vi "FlowThroughNMR.vi"() -> ()   [LabVIEW 2021]
uses:
  <instrlib>/niFgen/niFgen.llb/niFgen Output Mode.ctl
  <vilib>/Utility/file.llb/Write Delimited Spreadsheet (DBL).vi
panel:
  in  "File Folder for Data":string
  out "size(s)":i32
  out "Numeric":dbl
  in  "Write Output to File?":bool=TRUE
  out "Averaged T2 Decay":waveform(dbl)(graph)={"t0"=timestamp(0 s since 1904-01-01), "dt"=0.0012610340479192938, "Y"=array[3965 elements]} caption="Waveform Graph"
  in  "Number of Scans":i32=8
  out "Signal Intensity (Integral)":dbl=0.6544283602926818 format="%0.4f"
  out "Scan Number":i32=8
  out "Final Larmor Frequency":dbl format="%#_10g"
  in  "Pulse Train File":path=path "C:/Users/localuser/OneDrive - University of South Carolina/NMR Research/MATLAB/6 us 90 Degree - 1.25ms Tau - 3965 Pulses.txt"
  in  "Initial Larmor Frequency":dbl=27410000.0 caption="Frequency" format="%.3p"
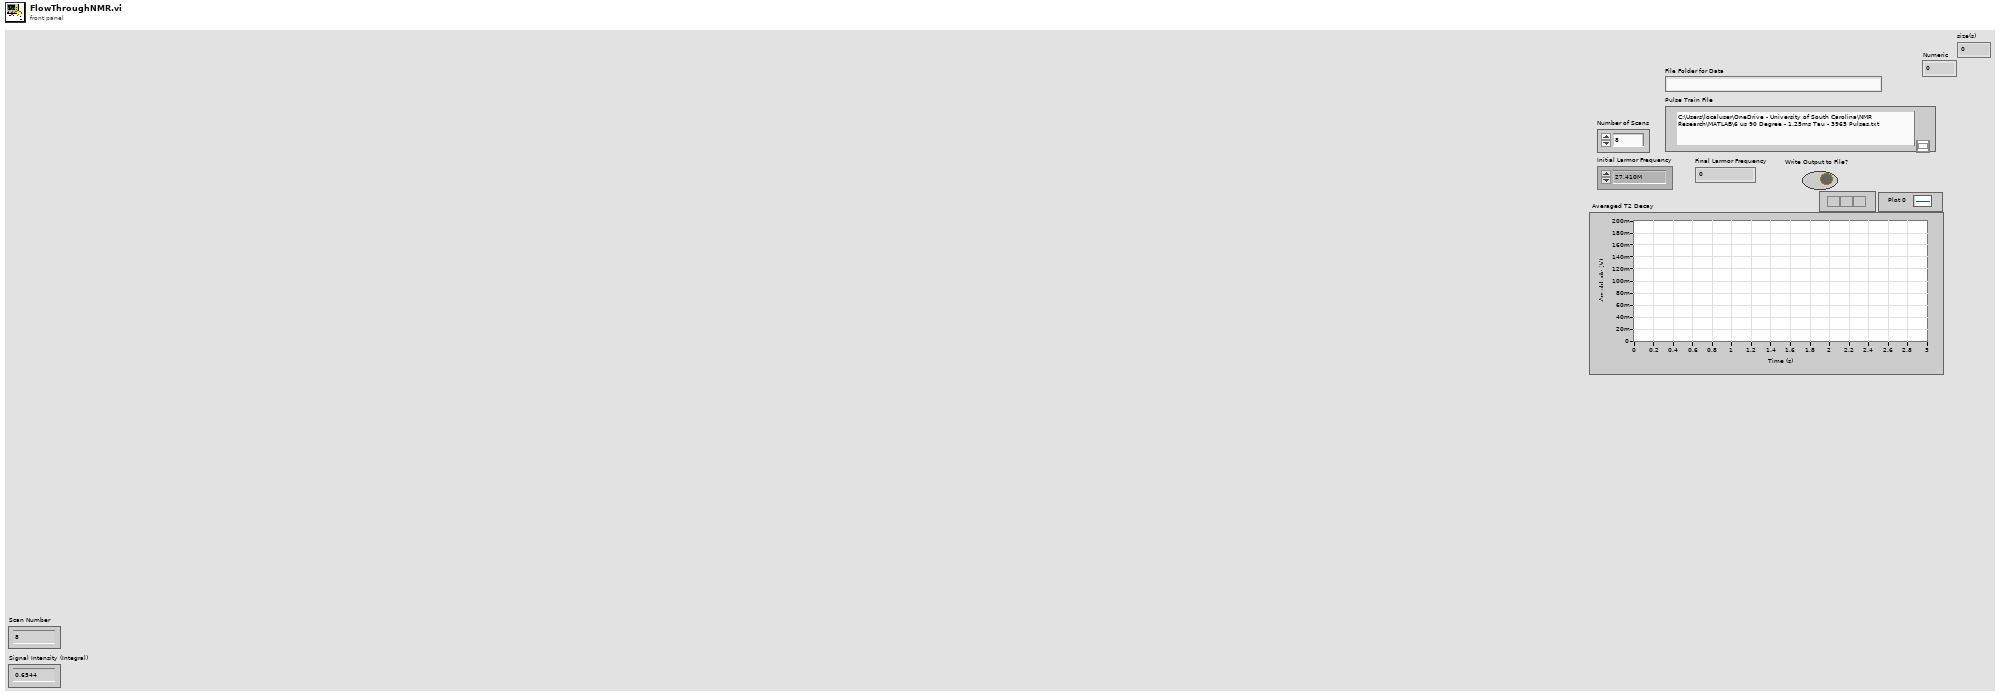
[diagram p1: front panel]
types:
  T1 = typedef "niFgen Output Mode.ctl" = u32
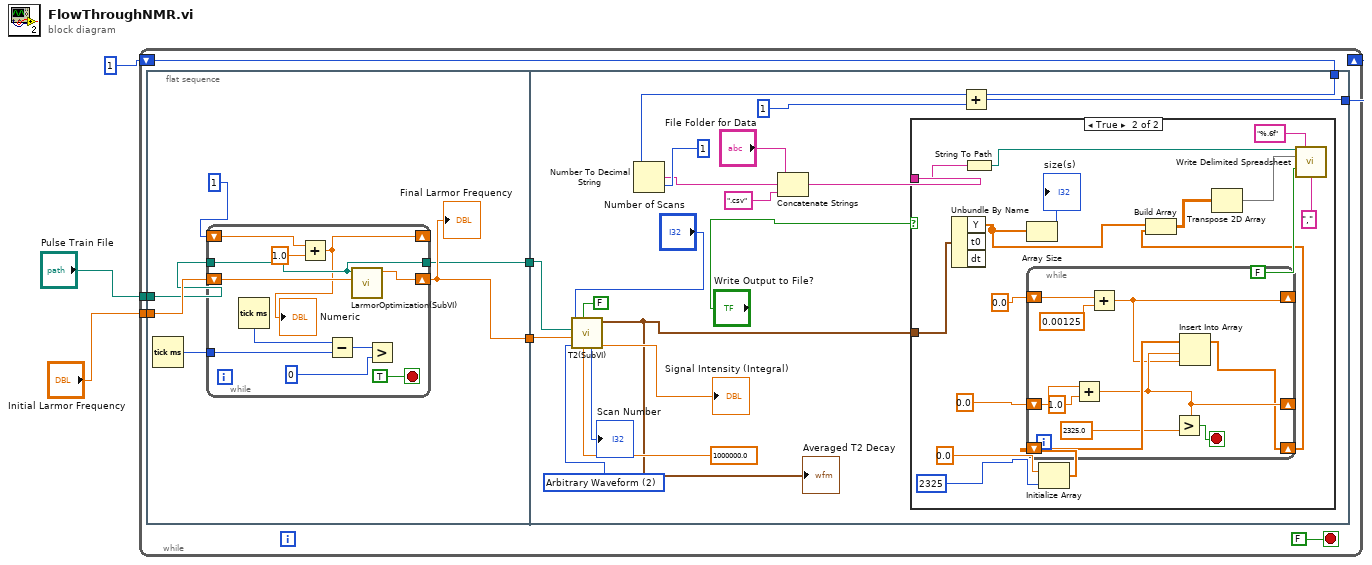
[diagram p0: block diagram]
diagram:
  n1 = while {
    tunnel: "Initial Larmor Frequency" -> [w10]
    tunnel: "Pulse Train File" -> [w9]
    shift-right: [w6] -> _
    shift-left: 1 -> [w7]
    stop <- FALSE stop-if-true
    n2 = flat-sequence {
      tunnel: w9 -> [w15]
      tunnel: w10 -> [w16]
      tunnel: [w13] -> w5
      tunnel: [w12] -> w4
      tunnel: w7 -> [w37]
      tunnel: [w35] -> w6
      tunnel: w5 -> [w34]
      tunnel: w4 -> [w33]
      frame #0 {
        n3 = Tick Count (ms)() -> (millisecond timer value=w14:u32)
        n4 = while {
          shift-right: [w27] -> w13
          shift-left: w16 -> [w26]
          tunnel: w15 -> [w21]
          tunnel: w14 -> [w23]
          tunnel: [w21] -> w12
          shift-right: [w18] -> _
          shift-left: 1 -> [w19]
          stop <- TRUE stop-if-true
          n5 = Tick Count (ms)() -> (millisecond timer value=w24:u32)
          n6 = Add(x=w19, y=1.0) -> (x+y=w18:dbl)
          "Numeric" <- w18
          n7 = Subtract(x=w24, y=w23) -> (x-y=w22:u32)
          n8 = call "LarmorOptimization(SubVI).vi"("Initial Larmor Frequency"=w26, "Pulse Train File in"=w21) -> ("Larmor Frequency 3"=w27:dbl)  [unwired: 9 in]
          n9 = Greater?(x=w22, y=u32 0) -> ()  [unwired: 1 out]
        }
        "Final Larmor Frequency" <- w13
      }
      frame #1 {
        w42 = T1 2 items=["Standard Function", "Frequency List", "Arbitrary Waveform", "Arbitrary Sequence", "Script"] ("output mode")
        n10 = call "T2(SubVI).vi"("Sample Rate"=1000000.0, "Write Output to File?"=FALSE, "output mode"=w42, "Larmor Frequency"=w34, "Pulse Train File"=w33, "Number of Scans"="Number of Scans") -> ("Signal Intensity (Integral)"=→"Signal Intensity (Integral)":dbl, "Averaged T2 Decay"=w29:waveform(dbl), "Scan Number"=→"Scan Number":i32)  [unwired: 3 out]
        "Averaged T2 Decay" <- w29
        n11 = Number To Decimal String(number=w37, width (-)=i16 1) -> (decimal integer string=w30:string)
        n12 = Concatenate Strings("File Folder for Data", w30, ".csv" ("string")) -> (w32:string)
        n13 = case shown="True" "Write Output to File?" {
          tunnel: w32 -> [_ w61]
          tunnel: w29 -> [_ w57]
          frame False {
          }
          frame True {
            n14 = Unbundle By Name(w57) -> ("Y"=w50:dbl[])  [unwired: 2 out]
            n15 = String To Path(string=w61) -> (path=w60:path)
            n16 = Array Size(array=w50) -> (size(s)=→"size(s)":i32)
            n17 = Initialize Array(0.0 ("element"), 2325 ("dimension size")) -> (w55:dbl[])
            n18 = while {
              shift-right: [w62] -> _
              shift-left: 0.0 -> [w69]
              shift-right: [w64] -> _
              shift-left: 0.0 -> [w65]
              shift-right: [w63] -> w49
              shift-left: w55 -> [w68]
              stop <- w67 stop-if-true
              n19 = Add(x=w65, y=1.0) -> (x+y=w64:dbl)
              n20 = Add(x=w69, y=0.00125) -> (x+y=w62:dbl)
              n21 = Greater?(x=w64, y=2325.0) -> (0:w67:bool)
              n22 = Insert Into Array(array=w68, index=w64, new element=w62) -> (w63:dbl[])
            }
            n23 = Build Array(w50, w49) -> (w48:dbl[][])
            n24 = Transpose 2D Array(2D array=w48) -> (transposed array=w47:dbl[][])
            n25 = call-poly <vilib>:"Write Delimited Spreadsheet.vi"("file path (dialog if empty)"=w60, "format (%.3f)"="%.6f", "2D data"=w47, "append to file? (new file:F)"=FALSE, "delimiter (\\t)"="," ("delimiter (\\t)")) -> ()  [unwired: 9 in, 2 out]
          }
        }
        n26 = Add(x=w37, y=1) -> (x+y=w35:i32)
      }
    }
  }
